vi "T2_meas_freq.vi"() -> ()   [LabVIEW 2014]
uses:
  <vilib>/Utility/file.llb/Write To Spreadsheet File (DBL).vi
  <vilib>/Utility/file.llb/Read From Spreadsheet File (DBL).vi
  <vilib>/gmath/NumericalOptimization/Nonlinear Curve Fit LM formula string.vi
  <vilib>/gmath/NI_Gmath.lvlib
  <vilib>/Analysis/NI_AALBase.lvlib
panel:
  in  "semester":string(combo)="ws17"
  in  "Y-range":dbl=10.0
  in  "X-range":dbl=120.0
  out "hlim":dbl=1124.3902439024391 format="%#.1f"
  out "llim":dbl=775.609756097561 format="%#.1f"
  out "spin echo\nsignal":dbl=39.43929300282765 format="%#.2g"
  in  "time-\n  out":u32=6
  in  "gain":u32=1000
  out "Fourier spectrum":cluster{"Y":dbl[], "Y":dbl[]}[](graph)
  in  "del T (+-)":u32=10
  in  "folder":string
  in  "don`t write data, update plot, no fit:":bool=TRUE
  out "init values:":dbl[](array[numeric])=[200.0, 20.0, 1e-05]
  out "error A":dbl[](array[numeric]) format="%#.1f"
  out "error T2[ms]":dbl[](array[numeric]) format="%#.1f"
  out "Tdiff":dbl[](array[numeric]) format="%#.1e"
  out "A":dbl[](array[numeric]) format="%#.1f"
  out "T2[ms]":dbl[](array[numeric]) format="%#.1f"
  in  "fit:":bool=TRUE
  out "XY Graph":cluster{"Y":dbl[], "Y":dbl[]}[](graph) caption="Data"
  out "error echo amplv":dbl[](array[numeric])=[0.2412723, 0.1805783] format="%.3f"
  out "echo amplv":dbl[](array[numeric])=[47.4269393, 39.0815663] format="%.2f"
  out "echo timev":dbl[](array[numeric])=[40.0000003, 80.0000003] format="%#.1f"
  in  "many measurements:":bool=TRUE
  out "x+y":i32=10
  in  "data file":string="test"
  out "error avg peak":dbl format="%.3f"
  out "avg peak":dbl format="%.2f"
  out "amplitude window":cluster{"Y":dbl[], "Y":dbl[]}[](graph)
  out "amplitude":cluster{"Y":dbl[], "Y":dbl[]}[](graph) caption="XY Graph"
  in  "scan freq [kHz]":u32=10
  in  "meas. time":u32=120
  in  "number meas":i32=10
  in  "spin echo time":u32=80
  in  "write data to file, update plot:":bool
  in  "single measurement:":bool=TRUE
  in  "stop":bool
  # "peak window"
  # "1)"
  # "2)"
  # "data measured:"
  # "3)"
  # "4)"
  # "A"
  # "5)"
  # "fit values:"
  # "T2[ms]"
  # "Tdiff"
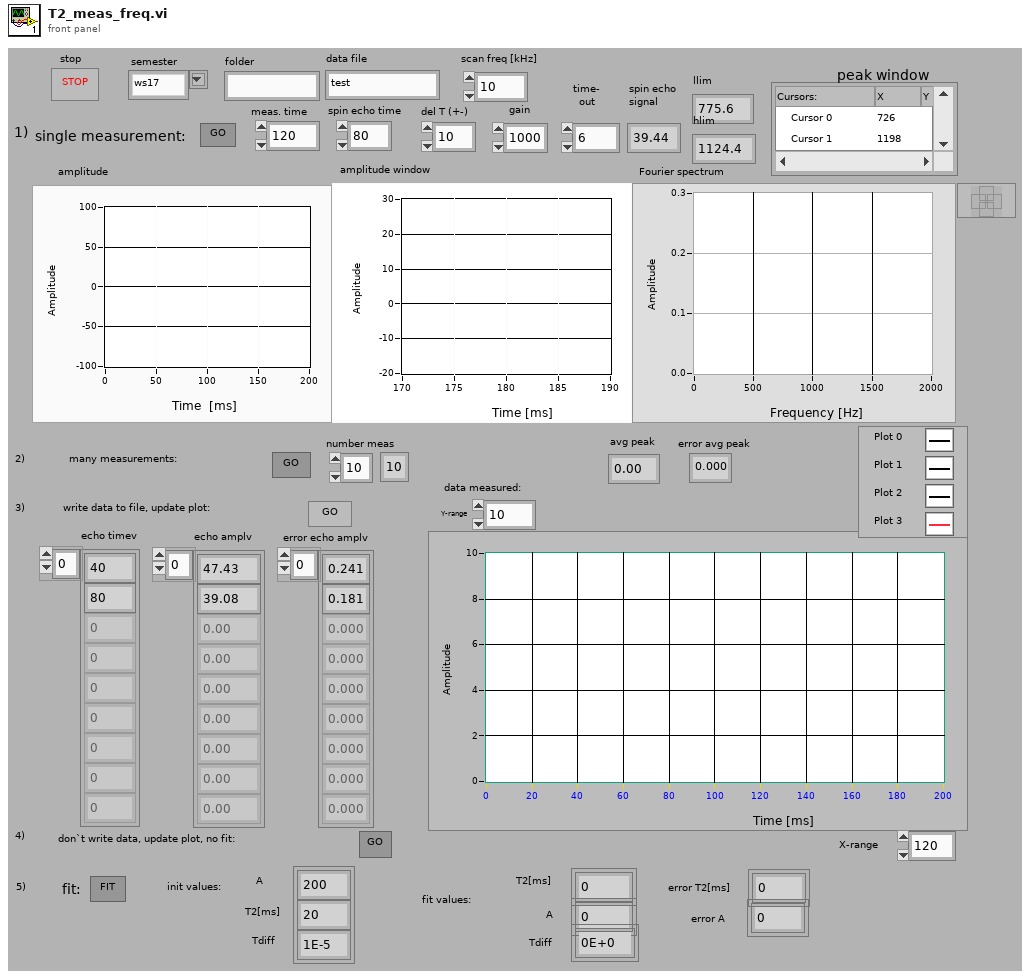
[diagram p1: front panel]
types:
  T1 = cluster{"model":string, "Parameters":string[], "x":string}
  T2 = typedef "LVCursorListTypeDef.ctl" = cluster{"Name":string, "Color":u32, "Style":u8, "Point Style":u8, "Name Visible":bool, "Allow Drag":bool, "Cursor Mode":u32, "Plot":i32, "Index":i32, "Position":cluster{"X":dbl, "Y":dbl}, "X Scale":u32, "Y Scale":u32, "Watch Plots":i32[], "Watch All Plots":bool, "Plot Area":i32, "Label Offset":cluster{"X":dbl, "Y":dbl}}[]
  T3 = typedef "NI_Matrix.lvlib/RealMatrix.ctl" = dbl[][]
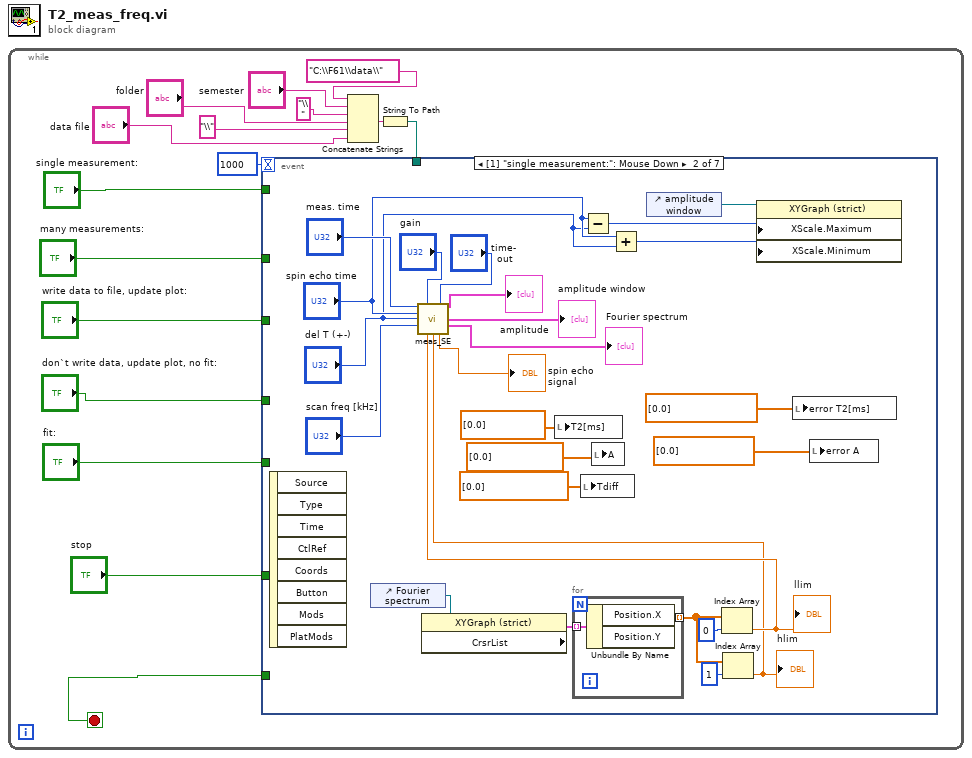
[diagram p0: block diagram]
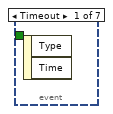
[diagram p2: hidden frame]
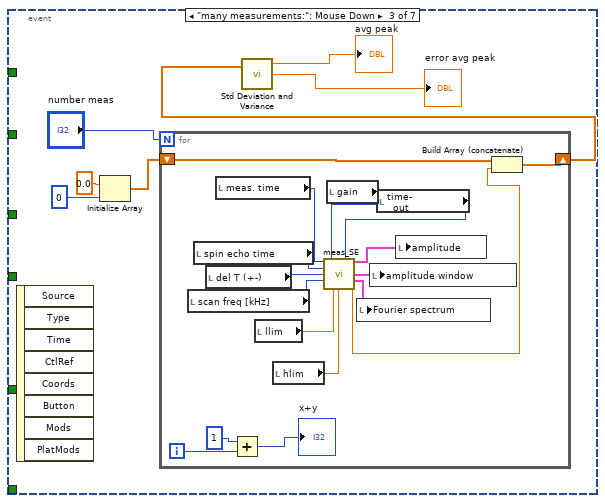
[diagram p3: hidden frame]
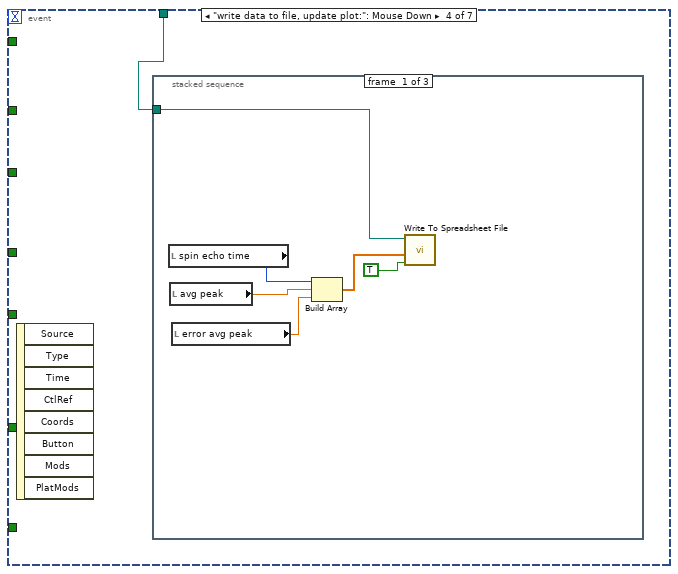
[diagram p4: hidden frame]
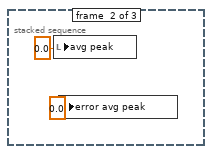
[diagram p5: hidden frame]
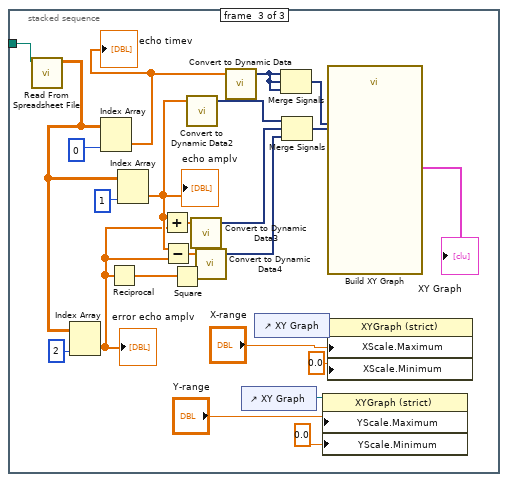
[diagram p6: hidden frame]
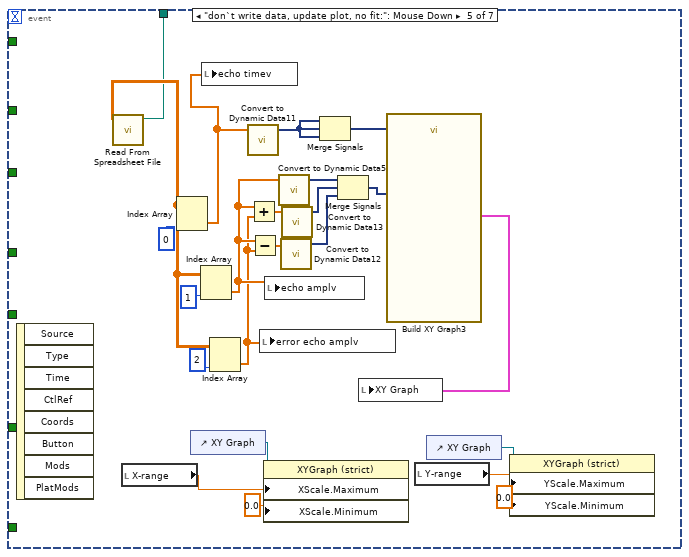
[diagram p7: hidden frame]
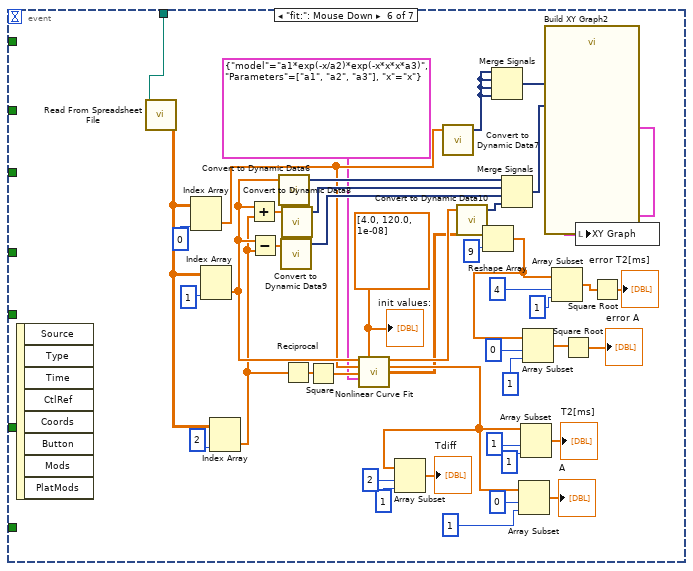
[diagram p8: hidden frame]
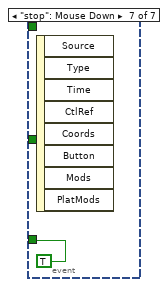
[diagram p9: hidden frame]
diagram:
  n1 = while {
    stop <- w9 stop-if-true
    n2 = Concatenate Strings("C:\\F61\\data\\", "semester", "\\" ("string"), "folder", "\\" ("string"), "data file") -> (w14:string)
    n3 = String To Path(string=w14) -> (path=w13:path)
    n4 = event shown="[1] \"single measurement:\": Mouse Down" {
      selector: _ -> [_ _ _ _ _ _ _]
      dyn-events: _ -> [_ _ _ _ _ _ _]
      timeout: 1000 -> [_ _ _ _ _ _ _]
      tunnel: "single measurement:" -> [_ _ _ _ _ _ _]
      tunnel: "write data to file, update plot:" -> [_ _ _ _ _ _ _]
      tunnel: w13 -> [_ _ _ w68 w112 w146 _]
      tunnel: "many measurements:" -> [_ _ _ _ _ _ _]
      tunnel: "fit:" -> [_ _ _ _ _ _ _]
      tunnel: "stop" -> [_ _ _ _ _ _ _]
      tunnel: [_ _ _ _ _ _ TRUE ("stop")] -> w9
      tunnel: "don`t write data, update plot, no fit:" -> [_ _ _ _ _ _ _]
      event Timeout {
        n5 = event-data() -> ()  [unwired: 1 in, 2 out]
      }
      event "single measurement:": Mouse Down {
        n6 = event-data() -> ()  [unwired: 1 in, 8 out]
        n7 = control-ref of="Fourier spectrum"() -> (w41:refnum<vi>)
        n8 = property class="XYGraph (strict)"(reference=w41) -> ("CrsrList"=w40:T2)  [unwired: 1 in, 2 out]
        n9 = local write "T2[ms]"(dbl[] [0.0] ("T2[ms]")) -> ()
        n10 = for {
          tunnel: w40 -> [w43] mode=indexing
          tunnel: [w42] -> w39 mode=indexing
          n11 = Unbundle By Name(w43) -> ("Position.X"=w42:dbl)  [unwired: 1 out]
        }
        n12 = local write "Tdiff"(dbl[] [0.0] ("Tdiff")) -> ()
        n13 = Subtract(x="spin echo time", y="del T (+-)") -> (x-y=w23:u32)
        n14 = local write "A"(dbl[] [0.0] ("A")) -> ()
        n15 = Add(x="spin echo time", y="del T (+-)") -> (x+y=w22:u32)
        n16 = control-ref of="amplitude window"() -> (w26:refnum<vi>)
        n17 = Index Array(array=w39, index=0) -> (element=w28:dbl)
        "llim" <- w28
        n18 = Index Array(array=w39, index=1) -> (element=w27:dbl)
        "hlim" <- w27
        n19 = call "meas_SE.vi"("meas. time [ms]"="meas. time", "gainfac"="gain", "time out [s]"="time-\n  out", "spin echo time [ms]"="spin echo time", "del T (+-) ][ms]"="del T (+-)", "scan freq [kHz]"="scan freq [kHz]", "llim"=w28, "hlim"=w27) -> ("Amplitude"=→"amplitude":cluster{"Y":dbl[], "Y":dbl[]}[], "Spin echo (time)"=→"amplitude window":cluster{"Y":dbl[], "Y":dbl[]}[], "Spin echo (freq)"=→"Fourier spectrum":cluster{"Y":dbl[], "Y":dbl[]}[], "SE-corr"=→"spin echo\nsignal":dbl)  [unwired: 3 in, 1 out]
        n20 = property class="XYGraph (strict)"(reference=w26, "XScale.Maximum"=w23, "XScale.Minimum"=w22) -> ()  [unwired: 1 in, 2 out]
        n21 = local write "error T2[ms]"(dbl[] [0.0] ("error T2[ms]")) -> ()
        n22 = local write "error A"(dbl[] [0.0] ("error A")) -> ()
      }
      event "many measurements:": Mouse Down {
        n23 = event-data() -> ()  [unwired: 1 in, 8 out]
        n24 = Initialize Array(0.0 ("element"), 0 ("dimension size")) -> (w48:dbl[])
        n25 = for {
          N: "number meas" -> [_]
          shift-right: [w63] -> w47
          shift-left: w48 -> [w64]
          i -> [w66]
          n26 = local read "scan freq [kHz]"() -> (w59:u32)
          n27 = local read "spin echo time"() -> (w61:u32)
          n28 = local read "del T (+-)"() -> (w60:u32)
          n29 = local read "meas. time"() -> (w62:u32)
          n30 = Add(x=1, y=w66) -> (x+y=→"x+y":i32)
          n31 = local read "llim"() -> (w55:dbl)
          n32 = local read "hlim"() -> (w54:dbl)
          n33 = local read "gain"() -> (w58:u32)
          n34 = local read "time-\n  out"() -> (w57:u32)
          n35 = call "meas_SE.vi"("meas. time [ms]"=w62, "gainfac"=w58, "time out [s]"=w57, "spin echo time [ms]"=w61, "del T (+-) ][ms]"=w60, "scan freq [kHz]"=w59, "llim"=w55, "hlim"=w54) -> ("Amplitude"=w53:cluster{"Y":dbl[], "Y":dbl[]}[], "Spin echo (time)"=w52:cluster{"Y":dbl[], "Y":dbl[]}[], "Spin echo (freq)"=w51:cluster{"Y":dbl[], "Y":dbl[]}[], "SE-corr"=w56:dbl)  [unwired: 3 in, 1 out]
          n36 = local write "Fourier spectrum"(w51) -> ()
          n37 = local write "amplitude window"(w52) -> ()
          n38 = local write "amplitude"(w53) -> ()
          n39 = Build Array (concatenate)(w64, w56) -> (w63:dbl[])
        }
        n40 = call <vilib>:"Std Deviation and Variance.vi"("X"=w47) -> ("mean"=→"avg peak":dbl, "standard deviation"=→"error avg peak":dbl)  [unwired: 1 in, 1 out]
      }
      event "write data to file, update plot:": Mouse Down {
        n41 = event-data() -> ()  [unwired: 1 in, 8 out]
        n42 = stacked-sequence {
          tunnel: w68 -> [w69 _ w100]
          frame #0 {
            n43 = local read "spin echo time"() -> (w70:u32)
            n44 = local read "avg peak"() -> (w71:dbl)
            n45 = local read "error avg peak"() -> (w74:dbl)
            n46 = Build Array(w70, w71, w74) -> (w72:dbl[])
            n47 = call-poly <vilib>:"Write To Spreadsheet File.vi"("append to file? (new file:F)"=TRUE, "1D data"=w72, "file path (dialog if empty)"=w69) -> ()  [unwired: 5 in, 1 out]
          }
          frame #1 {
            n48 = local write "avg peak"(sgl 0.0 ("avg diff")) -> ()
            n49 = local write "error avg peak"(0.0 ("error avg diff")) -> ()
          }
          frame #2 {
            n50 = call-poly <vilib>:"Read From Spreadsheet File.vi"("file path (dialog if empty)"=w100) -> ("all rows"=w99:dbl[][])  [unwired: 6 in, 4 out]
            n51 = Index Array(array=w99, index (col)=2 ("index (row)")) -> (element=w85:dbl[])  [unwired: 1 in]
            "error echo amplv" <- w85
            n52 = Index Array(array=w99, index (col)=0 ("index (row)")) -> (element=w83:dbl[])  [unwired: 1 in]
            "echo timev" <- w83
            n53 = Reciprocal(x=w85) -> (1/x=w84:dbl[])
            n54 = Index Array(array=w99, index (col)=1 ("index (row)")) -> (element=w86:dbl[])  [unwired: 1 in]
            "echo amplv" <- w86
            n55 = Add(x=w86, y=w85) -> (x+y=w90:dbl[])
            n56 = Subtract(x=w86, y=w85) -> (x-y=w89:dbl[])
            n57 = Square(x=w84) -> ()  [unwired: 1 out]
            n58 = call "Convert to Dynamic Data2"("Array"=w86) -> ("Dynamic Data Type"=w91:dynamicdata)  [unwired: 3 in]
            n59 = call "Convert to Dynamic Data3"("Array"=w90) -> ("Dynamic Data Type"=w88:dynamicdata)  [unwired: 3 in]
            n60 = call "Convert to Dynamic Data4"("Array"=w89) -> ("Dynamic Data Type"=w87:dynamicdata)  [unwired: 3 in]
            n61 = call "Convert to Dynamic Data"("Array"=w83) -> ("Dynamic Data Type"=w94:dynamicdata)  [unwired: 3 in]
            n62 = control-ref of="XY Graph"() -> (w79:refnum<vi>)
            n63 = control-ref of="XY Graph"() -> (w82:refnum<vi>)
            n64 = Merge Signals(w94, w94, w94) -> (w93:dynamicdata)
            n65 = Merge Signals(w91, w88, w87) -> (w92:dynamicdata)
            n66 = property class="XYGraph (strict)"(reference=w79, "YScale.Maximum"="Y-range", "YScale.Minimum"=0.0 ("Y Scale.Range:Maximum")) -> ()  [unwired: 1 in, 2 out]
            n67 = call "Build XY Graph"("Y Input"=w92, "X Input"=w93) -> ("XY Graph"=→"XY Graph":cluster{"Y":dbl[], "Y":dbl[]}[])  [unwired: 8 in, 1 out]
            n68 = property class="XYGraph (strict)"(reference=w82, "XScale.Maximum"="X-range", "XScale.Minimum"=0.0 ("X Scale.Range:Maximum")) -> ()  [unwired: 1 in, 2 out]
          }
        }
      }
      event "don`t write data, update plot, no fit:": Mouse Down {
        n69 = event-data() -> ()  [unwired: 1 in, 8 out]
        n70 = call-poly <vilib>:"Read From Spreadsheet File.vi"("file path (dialog if empty)"=w112) -> ("all rows"=w123:dbl[][])  [unwired: 6 in, 4 out]
        n71 = local read "X-range"() -> (w105:dbl)
        n72 = Index Array(array=w123, index (col)=0 ("index (row)")) -> (element=w109:dbl[])  [unwired: 1 in]
        n73 = control-ref of="XY Graph"() -> (w104:refnum<vi>)
        n74 = Index Array(array=w123, index (col)=1 ("index (row)")) -> (element=w108:dbl[])  [unwired: 1 in]
        n75 = local write "echo timev"(w109) -> ()
        n76 = Index Array(array=w123, index (col)=2 ("index (row)")) -> (element=w107:dbl[])  [unwired: 1 in]
        n77 = call "Convert to Dynamic Data11"("Array"=w109) -> ("Dynamic Data Type"=w110:dynamicdata)  [unwired: 3 in]
        n78 = Add(x=w108, y=w107) -> (x+y=w116:dbl[])
        n79 = Subtract(x=w108, y=w107) -> (x-y=w115:dbl[])
        n80 = local write "error echo amplv"(w107) -> ()
        n81 = property on="Property Node" class="XYGraph (strict)"(reference=w104, "XScale.Maximum"=w105, "XScale.Minimum"=0.0 ("X Scale.Range:Maximum")) -> ()  [unwired: 1 in, 2 out]
        n82 = local write "echo amplv"(w108) -> ()
        n83 = call "Convert to Dynamic Data5"("Array"=w108) -> ("Dynamic Data Type"=w117:dynamicdata)  [unwired: 3 in]
        n84 = call "Convert to Dynamic Data12"("Array"=w115) -> ("Dynamic Data Type"=w113:dynamicdata)  [unwired: 3 in]
        n85 = call "Convert to Dynamic Data13"("Array"=w116) -> ("Dynamic Data Type"=w114:dynamicdata)  [unwired: 3 in]
        n86 = Merge Signals(w110, w110, w110) -> (w119:dynamicdata)
        n87 = Merge Signals(w117, w114, w113) -> (w118:dynamicdata)
        n88 = call "Build XY Graph3"("Y Input"=w118, "X Input"=w119) -> ("XY Graph"=w111:cluster{"Y":dbl[], "Y":dbl[]}[])  [unwired: 8 in, 1 out]
        n89 = local write "XY Graph"(w111) -> ()
        n90 = local read "Y-range"() -> (w101:dbl)
        n91 = control-ref of="XY Graph"() -> (w103:refnum<vi>)
        n92 = property class="XYGraph (strict)"(reference=w103, "YScale.Maximum"=w101, "YScale.Minimum"=0.0 ("Y Scale.Range:Minimum")) -> ()  [unwired: 1 in, 2 out]
      }
      event "fit:": Mouse Down {
        w124 = dbl[] [4.0, 120.0, 1e-08] ("init values")
        n93 = event-data() -> ()  [unwired: 1 in, 8 out]
        n94 = call-poly <vilib>:"Read From Spreadsheet File.vi"("file path (dialog if empty)"=w146) -> ("all rows"=w167:dbl[][])  [unwired: 6 in, 4 out]
        n95 = Index Array(array=w167, index (col)=0 ("index (row)")) -> (element=w150:dbl[])  [unwired: 1 in]
        n96 = Index Array(array=w167, index (col)=1 ("index (row)")) -> (element=w156:dbl[])  [unwired: 1 in]
        n97 = Index Array(array=w167, index (col)=2 ("index (row)")) -> (element=w155:dbl[])  [unwired: 1 in]
        n98 = Add(x=w156, y=w155) -> (x+y=w160:dbl[])
        n99 = Subtract(x=w156, y=w155) -> (x-y=w159:dbl[])
        n100 = call "Convert to Dynamic Data6"("Array"=w156) -> ("Dynamic Data Type"=w161:dynamicdata)  [unwired: 3 in]
        n101 = call "Convert to Dynamic Data9"("Array"=w159) -> ("Dynamic Data Type"=w157:dynamicdata)  [unwired: 3 in]
        n102 = call "Convert to Dynamic Data8"("Array"=w160) -> ("Dynamic Data Type"=w158:dynamicdata)  [unwired: 3 in]
        n103 = Reciprocal(x=w155) -> (1/x=w154:dbl[])
        n104 = Square(x=w154) -> (x^2=w153:dbl[])
        n105 = call-poly <vilib>:"Nonlinear Curve Fit.vi"("Y"=w156, "initial parameters"=w124, "X"=w150, "Weight"=w153, "model description"=T1 {"model"="a1*exp(-x/a2)*exp(-x*x*x*a3)", "Parameters"=["a1", "a2", "a3"], "x"="x"}) -> ("best nonlinear fit"=w152:dbl[], "best fit parameters"=w139:dbl[], "covariance"=w136:T3)  [unwired: 6 in, 2 out]
        n106 = Array Subset(array=w139, index=2, length=1) -> (→"Tdiff":dbl[])
        n107 = call "Convert to Dynamic Data7"("Array"=w150) -> ("Dynamic Data Type"=w131:dynamicdata)  [unwired: 3 in]
        n108 = call "Convert to Dynamic Data10"("Array"=w152) -> ("Dynamic Data Type"=w151:dynamicdata)  [unwired: 3 in]
        n109 = Reshape Array(w136, 9 ("dimension size")) -> (w126:dbl[])
        n110 = Merge Signals(w131, w131, w131, w131) -> (w163:dynamicdata)
        n111 = Merge Signals(w161, w158, w157, w151) -> (w162:dynamicdata)
        n112 = Array Subset(array=w139, index=0, length=1) -> (→"A":dbl[])
        n113 = Array Subset(array=w139, index=1, length=1) -> (→"T2[ms]":dbl[])
        n114 = Array Subset(array=w126, index=0, length=1 ("index")) -> (w127:dbl[])
        n115 = call "Build XY Graph2"("Y Input"=w162, "X Input"=w163) -> ("XY Graph"=w144:cluster{"Y":dbl[], "Y":dbl[]}[])  [unwired: 8 in, 1 out]
        n116 = Array Subset(array=w126, index=4, length=1 ("index")) -> (w132:dbl[])
        n117 = Square Root(x=w127) -> (sqrt(x)=→"error A":dbl[])
        n118 = local write "XY Graph"(w144) -> ()
        n119 = Square Root(x=w132) -> (sqrt(x)=→"error T2[ms]":dbl[])
        "init values:" <- w124
      }
      event "stop": Mouse Down {
        n120 = event-data() -> ()  [unwired: 1 in, 8 out]
      }
    }
  }
